vi "Framework Test.vi"() -> ()   [LabVIEW 2017]
uses:
  Source/Engine/Classes/Framework/DSF.Engine.Framework.lvclass
  <vilib>/platform/TimedLoop/XDataNode/XDataNode.xnode
  <vilib>/Platform/TimedLoop/XDataNode/nitl_modes.ctl
  <vilib>/Platform/TimedLoop/XDataNode/XDNodeRunTimeDep.lvlib
  <vilib>/Platform/TimedLoop/XDataNode/wakeup.ctl
  <vilib>/Platform/TimedLoop/XDataNode/timing_clust.ctl
  <vilib>/National Instruments/Memory Manager/Classes/Pointer/Memory.Pointer.lvclass
  <vilib>/National Instruments/Memory Manager/Classes/Pointer/Memory.Pointer.Write.0D.Bool.vi
  <vilib>/National Instruments/Memory Manager/Classes/Pointer/Memory.Pointer.New.4B.vi
  <vilib>/National Instruments/Memory Manager/Classes/Pointer/Memory.Pointer.Write.0D.U32.vi
  <vilib>/National Instruments/Memory Manager/Classes/Pointer/Memory.Pointer.Read.0D.U32.vi
  <vilib>/National Instruments/Memory Manager/Classes/Pointer/Memory.Pointer.Read.0D.Bool.vi
  <vilib>/National Instruments/Memory Manager/Classes/Pointer/Memory.Pointer.Write.0D.I32.vi
  <vilib>/National Instruments/Memory Manager/Classes/Pointer/Memory.Pointer.Read.0D.I32.vi
  <vilib>/National Instruments/Memory Manager/Classes/Pointer/Memory.Pointer.New.1B.vi
  Source/Plugins/Reflective Memory/DSF.Transceiver.GE Reflective Memory.lvclass
  Source/Plugins/PXImc/DSF.Transceiver.PXImc.lvclass
  Source/Plugins/UDP/DSF.Transceiver.UDP.lvclass
panel:
  out "Framework Iteration":i32 format="%d cycles"
  out "Actual Period":u32 format="%d us"
  in  "Target Period":u32=1000 format="%d us"
  in  "stop":bool
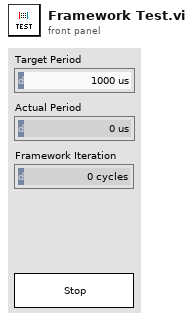
[diagram p1: front panel]
types:
  T1 = typedef "XDNodeRunTimeDep.lvlib/timing_clust.ctl" = cluster{"Expected End [f-1]":u64, "Actual End [f-1]":u64, "Finished Late? [f-1]":bool, "Expected End [i-1]":u64, "Actual End [i-1]":u64, "Finished Late? [i-1]":bool, "Expected Start [i]":u64, "Actual Start [i]":u64, "Expected Start [f]":u64, "Actual Start [f]":u64, "Source Name":string, "Structure Name":string, "Period":i64, "Deadline":i64, "Offset":i64, "Start":i64, "Priority":i32, "Timeout":i32, "Mode":T2, "Wakeup Reason":T3, "Error":errorcluster, "Source Type":string, "Secondary Source Type":string, "Global End Time":u64, "Global Start Time":u64, "Frame Duration":u64, "Iteration Duration":u64, "Assigned CPU":i32, "I/O Scan Engine Mode":u32}
  T2 = typedef "XDNodeRunTimeDep.lvlib/nitl_modes.ctl" = enum32{"No Change", "Process missed periods, maintain original phase", "Discard missed periods, maintain original phase", "Process missed periods, ignore original phase", "Discard missed periods, ignore original phase"}
  T3 = typedef "XDNodeRunTimeDep.lvlib/wakeup.ctl" = enum32{"Normal", "Aborted", "Asynchronous wakeup", "Timing source error", "Timed loop error", "Timeout"}
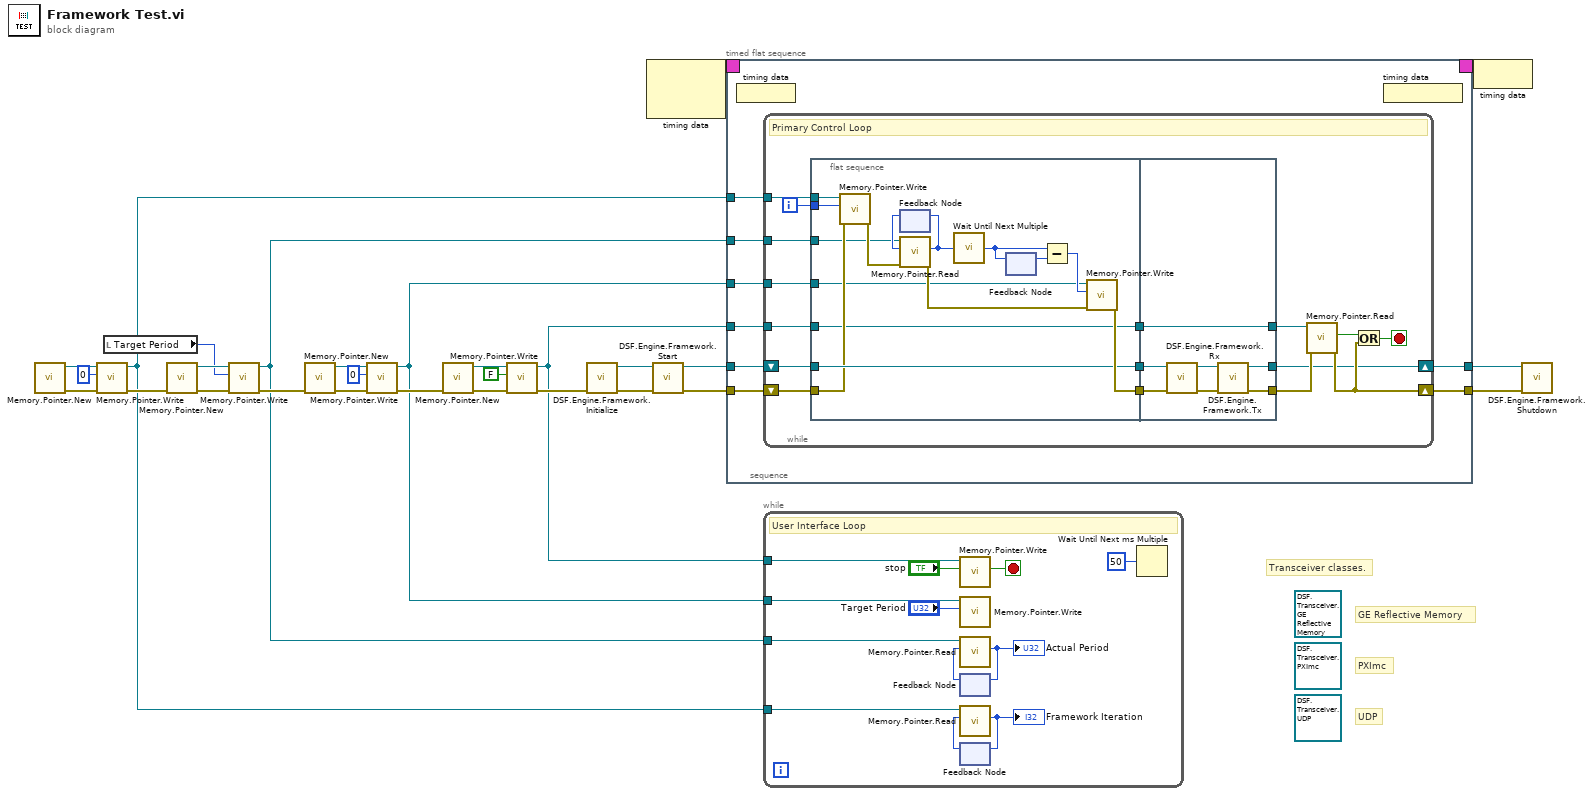
[diagram p0: block diagram]
diagram:
  (unwired) refnum<class "DSF.Transceiver.UDP.lvclass"> refnum ("DSF UDP Transceiver")
  (unwired) refnum<class "DSF.Transceiver.PXImc.lvclass"> refnum ("DSF PXImc Transceiver")
  (unwired) refnum<class "DSF.Transceiver.GE Reflective Memory.lvclass"> refnum ("DSF GE Reflective Memory Transceiver")
  # "Transceiver classes."
  # "UDP"
  # "PXImc"
  # "GE Reflective Memory"
  n1 = call-poly <vilib>:"Memory.Pointer.New.vi"() -> ("error out"=w5:errorcluster, "Pointer"=w7:refnum<class "Memory.Pointer.lvclass">)  [unwired: 10 in]
  n2 = call-poly <vilib>:"Memory.Pointer.Write.vi"("error in (no error)"=w5, "value"=u32 0, "Pointer in"=w7) -> ("error out"=w4:errorcluster, "Pointer out"=w1:refnum<class "Memory.Pointer.lvclass">)  [unwired: 5 in, 2 out]
  n3 = local read "Target Period"() -> (w15:u32)
  n4 = call-poly <vilib>:"Memory.Pointer.New.vi"("error in (no error)"=w4) -> ("error out"=w14:errorcluster, "Pointer"=w16:refnum<class "Memory.Pointer.lvclass">)  [unwired: 9 in]
  n5 = call-poly <vilib>:"Memory.Pointer.Write.vi"("error in (no error)"=w14, "value"=w15, "Pointer in"=w16) -> ("error out"=w13:errorcluster, "Pointer out"=w8:refnum<class "Memory.Pointer.lvclass">)  [unwired: 5 in, 2 out]
  n6 = call-poly <vilib>:"Memory.Pointer.New.vi"("error in (no error)"=w13) -> ("error out"=w11:errorcluster, "Pointer"=w17:refnum<class "Memory.Pointer.lvclass">)  [unwired: 9 in]
  n7 = call-poly <vilib>:"Memory.Pointer.Write.vi"("error in (no error)"=w11, "value"=u32 0, "Pointer in"=w17) -> ("error out"=w10:errorcluster, "Pointer out"=w9:refnum<class "Memory.Pointer.lvclass">)  [unwired: 5 in, 2 out]
  n8 = call-poly <vilib>:"Memory.Pointer.New.vi"("error in (no error)"=w10) -> ("error out"=w20:errorcluster, "Pointer"=w19:refnum<class "Memory.Pointer.lvclass">)  [unwired: 9 in]
  n9 = call-poly <vilib>:"Memory.Pointer.Write.vi"("error in (no error)"=w20, "value"=FALSE, "Pointer in"=w19) -> ("error out"=w3:errorcluster, "Pointer out"=w2:refnum<class "Memory.Pointer.lvclass">)  [unwired: 5 in, 2 out]
  n10 = call "DSF.Engine.Framework.Initialize.vi"("error in (no error)"=w3) -> ("error out"=w27:errorcluster, "Framework out"=w28:refnum<class "DSF.Engine.Framework.lvclass">)  [unwired: 9 in]
  n11 = node-c288() -> (w22:T1)  [unwired: 2 in]
  n12 = call "DSF.Engine.Framework.Start.vi"("error in (no error)"=w27, "Framework in"=w28) -> ("error out"=w25:errorcluster, "Framework out"=w26:refnum<class "DSF.Engine.Framework.lvclass">)  [unwired: 8 in]
  n13 = timed-sequence {
    timing: w22 -> [_]
    timing-out: [_] -> w21
    tunnel: w26 -> [w36]
    tunnel: w25 -> [w35]
    tunnel: [w34] -> w24
    tunnel: [w33] -> w23
    tunnel: w2 -> [w32]
    tunnel: w8 -> [w31]
    tunnel: w9 -> [w30]
    tunnel: w1 -> [w29]
    n14 = timed-flat-sequence {
      tunnel: w36 -> [w44]
      tunnel: w35 -> [w43]
      tunnel: [w42] -> w34
      tunnel: [w41] -> w33
      tunnel: w32 -> [w40]
      tunnel: w31 -> [w39]
      tunnel: w30 -> [w38]
      tunnel: w29 -> [w37]
      n15 = node-c288() -> ()  [unwired: 1 in]
      n16 = while {
        shift-right: [w47] -> w42
        shift-left: w44 -> [w59]
        shift-right: [w49] -> w41
        shift-left: w43 -> [w60]
        tunnel: w40 -> [w58]
        tunnel: w39 -> [w53]
        tunnel: w38 -> [w52]
        tunnel: w37 -> [w46]
        i -> [w45]
        stop <- w48 stop-if-true
        # "Primary Control Loop"
        n17 = flat-sequence {
          tunnel: w60 -> [w65]
          tunnel: w59 -> [w71]
          tunnel: w58 -> [w61]
          tunnel: [w72] -> w56
          tunnel: [w71] -> w55
          tunnel: [w61] -> w54
          tunnel: w53 -> [w63]
          tunnel: w52 -> [w62]
          tunnel: w46 -> [w67]
          tunnel: w45 -> [w66]
          tunnel: [w82] -> w57
          tunnel: w56 -> [w78]
          tunnel: w55 -> [w79]
          tunnel: w54 -> [w82]
          tunnel: [w77] -> w47
          tunnel: [w76] -> w51
          frame #0 {
            n18 = call-poly <vilib>:"Memory.Pointer.Write.vi"("error in (no error)"=w65, "value"=w66, "Pointer in"=w67) -> ("error out"=w64:errorcluster)  [unwired: 5 in, 3 out]
            n19 = feedback #1() -> (w69:u32)  [unwired: 1 in]
            n20 = call-poly <vilib>:"Memory.Pointer.Read.vi"("error in (no error)"=w64, "value in"=w69, "Pointer in"=w63) -> ("error out"=w68:errorcluster, "value out"=w70:u32)  [unwired: 5 in, 2 out]
            n21 = feedback-in #1(w70) -> ()
            n22 = call "Wait Until Next Multiple"("Count(uSec)"=w70) -> ("Tick Count(uSec)"=w75:u32)
            n23 = feedback #2() -> (w74:u32)  [unwired: 1 in]
            n24 = feedback-in #2(w75) -> ()
            n25 = Subtract(x=w75, y=w74) -> (x-y=w73:u32)
            n26 = call-poly <vilib>:"Memory.Pointer.Write.vi"("error in (no error)"=w68, "value"=w73, "Pointer in"=w62) -> ("error out"=w72:errorcluster)  [unwired: 5 in, 3 out]
          }
          frame #1 {
            n27 = call "DSF.Engine.Framework.Rx.vi"("error in (no error)"=w78, "Framework in"=w79) -> ("error out"=w81:errorcluster, "Framework out"=w80:refnum<class "DSF.Engine.Framework.lvclass">)  [unwired: 8 in]
            n28 = call "DSF.Engine.Framework.Tx.vi"("error in (no error)"=w81, "Framework in"=w80) -> ("error out"=w76:errorcluster, "Framework out"=w77:refnum<class "DSF.Engine.Framework.lvclass">)  [unwired: 8 in]
          }
        }
        n29 = call-poly <vilib>:"Memory.Pointer.Read.vi"("error in (no error)"=w51, "Pointer in"=w57) -> ("error out"=w49:errorcluster, "value out"=w50:bool)  [unwired: 6 in, 2 out]
        n30 = Or(x=w50, y=w49) -> (x .or. y?=w48:bool)
      }
      n31 = node-c288() -> ()  [unwired: 1 out]
    }
  }
  n32 = while {
    tunnel: w2 -> [w95]
    tunnel: w9 -> [w91]
    tunnel: w8 -> [w90]
    tunnel: w1 -> [w85]
    stop <- w96 stop-if-true
    # "User Interface Loop"
    n33 = call-poly <vilib>:"Memory.Pointer.Write.vi"("value"="stop", "Pointer in"=w95) -> ("value"=w96:bool)  [unwired: 6 in, 3 out]
    n34 = call-poly <vilib>:"Memory.Pointer.Write.vi"("value"="Target Period", "Pointer in"=w91) -> ()  [unwired: 6 in, 4 out]
    n35 = feedback #3() -> (w89:u32)  [unwired: 1 in]
    n36 = call-poly <vilib>:"Memory.Pointer.Read.vi"("value in"=w89, "Pointer in"=w90) -> ("value out"=w88:u32)  [unwired: 6 in, 3 out]
    "Actual Period" <- w88
    n37 = feedback-in #3(w88) -> ()
    n38 = feedback #4() -> (w86:i32)  [unwired: 1 in]
    n39 = call-poly <vilib>:"Memory.Pointer.Read.vi"("value in"=w86, "Pointer in"=w85) -> ("value out"=w87:i32)  [unwired: 6 in, 3 out]
    "Framework Iteration" <- w87
    n40 = feedback-in #4(w87) -> ()
    n41 = Wait Until Next ms Multiple(millisecond multiple=u32 50 ("milliseconds to wait")) -> ()  [unwired: 1 out]
  }
  n42 = node-c288(w21) -> ()
  n43 = call "DSF.Engine.Framework.Shutdown.vi"("error in (no error)"=w23, "Framework in"=w24) -> ()  [unwired: 8 in, 2 out]
